vi "shutdown timing source.vi"(8 "error in":errorcluster, 11 "timing source in":refnum<class "TBM timing source.lvclass">) -> (0 "error out":errorcluster, 3 "timing source out":refnum<class "TBM timing source.lvclass">)   [LabVIEW 2013, in "TBM timing source.lvclass"]
doc: "Shuts down the timing source. If a single timing source object is to be used as part of a loop which will be called multiple times, the best practice is to intialize the timing source prior to entering the loop and shutting the timing source down after exiting the loop. This may not be necessary if the selected timing source is stateless."
uses:
  TBM timing source.lvclass
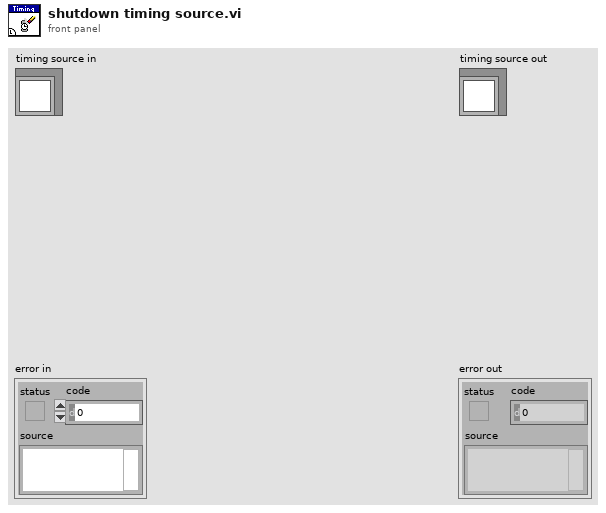
[diagram p1: front panel]
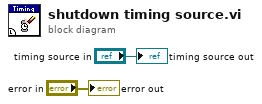
[diagram p0: block diagram]
diagram:
  "error out" <- "error in"
  "timing source out" <- "timing source in"
